vi "采水流程.vi"(11 "参数":T1) -> ()   [LabVIEW 2016]
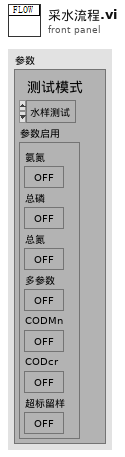
[diagram p1: front panel]
types:
  T1 = cluster{"测试模式":enum16{"水样测试", "平行样测试", "集成干预测试", "加标回收"}, "参数启用":cluster{"氨氮":bool, "总磷":bool, "总氮":bool, "多参数":bool, "CODMn":bool, "CODcr":bool, "超标留样":bool}}
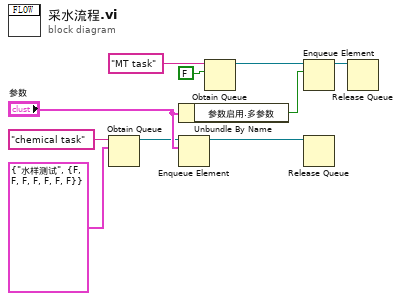
[diagram p0: block diagram]
diagram:
  n1 = Obtain Queue(name (unnamed)="chemical task" ("名称（未命名）"), element data type=T1 {"测试模式"=enum."水样测试", "参数启用"={"氨氮"=FALSE, "总磷"=FALSE, "总氮"=FALSE, "多参数"=FALSE, "CODMn"=FALSE, "CODcr"=FALSE, "超标留样"=FALSE}} ("参数")) -> (queue out=w5:refnum<queue>)  [unwired: 3 in, 2 out]
  n2 = Unbundle By Name("参数") -> ("参数启用.多参数"=w4:bool)
  n3 = Enqueue Element(queue=w5, element="参数") -> (queue out=w3:refnum<queue>)  [unwired: 2 in, 2 out]
  n4 = Obtain Queue(name (unnamed)="MT task" ("名称（未命名）"), element data type=FALSE) -> (queue out=w7:refnum<queue>)  [unwired: 3 in, 2 out]
  n5 = Enqueue Element(queue=w7, element=w4) -> (queue out=w2:refnum<queue>)  [unwired: 2 in, 2 out]
  n6 = Release Queue(queue=w3) -> ()  [unwired: 2 in, 3 out]
  n7 = Release Queue(queue=w2) -> ()  [unwired: 2 in, 3 out]
